vi "1WIRE_wait for convert.vi"(8 "error in":errorcluster) -> (0 "error out":errorcluster, 3 "Convert Time (usec)":u32)   [LabVIEW 2013]
doc: "This VI is created by Vincent Claes for FPDA-1 more information on http://pwo.fpga.be\n\nvincent.claes@xios.be\nclaesvincent@gmail.com\n\nhttp://www.linkedin.com/in/vincentclaes"
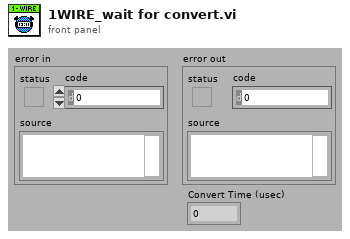
[diagram p1: front panel]
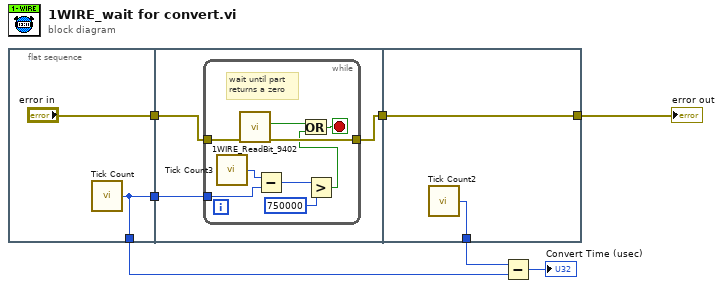
[diagram p0: block diagram]
diagram:
  n1 = flat-sequence {
    tunnel: ["error in"] -> w6
    tunnel: [w8] -> w3
    tunnel: [w8] -> w1
    tunnel: w6 -> [w12]
    tunnel: [w11] -> w5
    tunnel: w1 -> [w10]
    tunnel: [w23] -> w7
    tunnel: w5 -> [w23]
    tunnel: [w22] -> w4
    frame #0 {
      n2 = call "Tick Count"() -> ("Tick Count(uSec)"=w8:u32)
    }
    frame #1 {
      n3 = while {
        tunnel: w12 -> [w21]
        tunnel: [w19] -> w11
        tunnel: w10 -> [w17]
        stop <- w16 stop-if-true
        # "wait until part\nreturns a zero"
        n4 = call "Tick Count3"() -> ("Tick Count(uSec)"=w18:u32)
        n5 = call "1WIRE_ReadBit_9402.vi"("error in"=w21) -> ("error out"=w19:errorcluster, "Bit Read"=w20:bool)  [unwired: 9 in]
        n6 = Subtract(x=w18, y=w17) -> (x-y=w14:u32)
        n7 = Greater?(x=w14, y=u32 750000 ("x")) -> (0:w15:bool)
        n8 = Or(x=w20, y=w15) -> (x .or. y?=w16:bool)
      }
    }
    frame #2 {
      n9 = call "Tick Count2"() -> ("Tick Count(uSec)"=w22:u32)
    }
  }
  n10 = Subtract(x=w4, y=w3) -> (x-y=→"Convert Time (usec)":u32)
  "error out" <- w7
